vi "LIEF Example 4 - Main.vi"() -> ()   [LabVIEW 2017]
uses:
  Handler 4/Handler 4.lvclass
  C:/Program Files (x86)/National Instruments/LabVIEW 2017/vi.lib/LIEF/Image Editor Handler/Image Editor Handler.lvclass
  Cible/Cible.lvclass
  C:/Github/LIEF-Examples/LIEF Example4 - Drag&Drop/Circle/Circle.lvclass
  C:/Program Files (x86)/National Instruments/LabVIEW 2017/vi.lib/LIEF/Forms/Shape/Shape.lvclass
  <vilib>/LIEF/Image Editor Handler/Image Editor Handler.lvclass
  Circle/Circle.lvclass
  <vilib>/LIEF/Forms/Shape/Shape.lvclass
panel:
  in  "Del":bool
  in  "Boolean":bool
  out "Array":cluster{"Left":i32, "Top":i32}[](array[cluster])
  in  "Position":cluster{"Left":i32, "Top":i32}={"Left"=32, "Top"=32}
  out "Forms":picture[](array[picture])=[bytes[42], bytes[42], bytes[42], bytes[42], bytes[42], bytes[42], bytes[42], bytes[42], bytes[42], bytes[42]]
  in  "Scene":picture
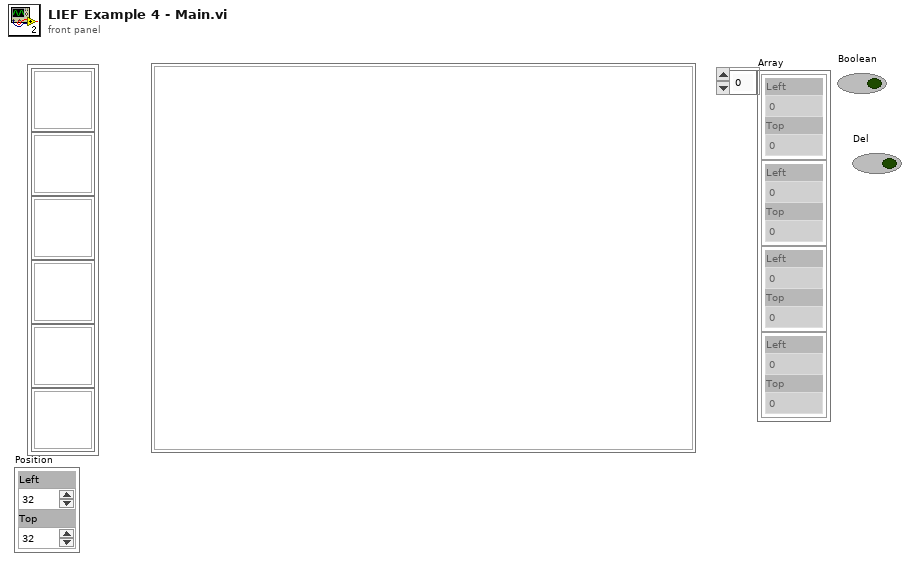
[diagram p1: front panel]
types:
  T1 = typedef "LVPoint32TypeDef.ctl" = cluster{"Horizontal":i32, "Vertical":i32}
  T2 = typedef "LVPositionTypeDef.ctl" = cluster{"Left":i32, "Top":i32}
  T3 = cluster{"data name":string, "drag data":variant}[]
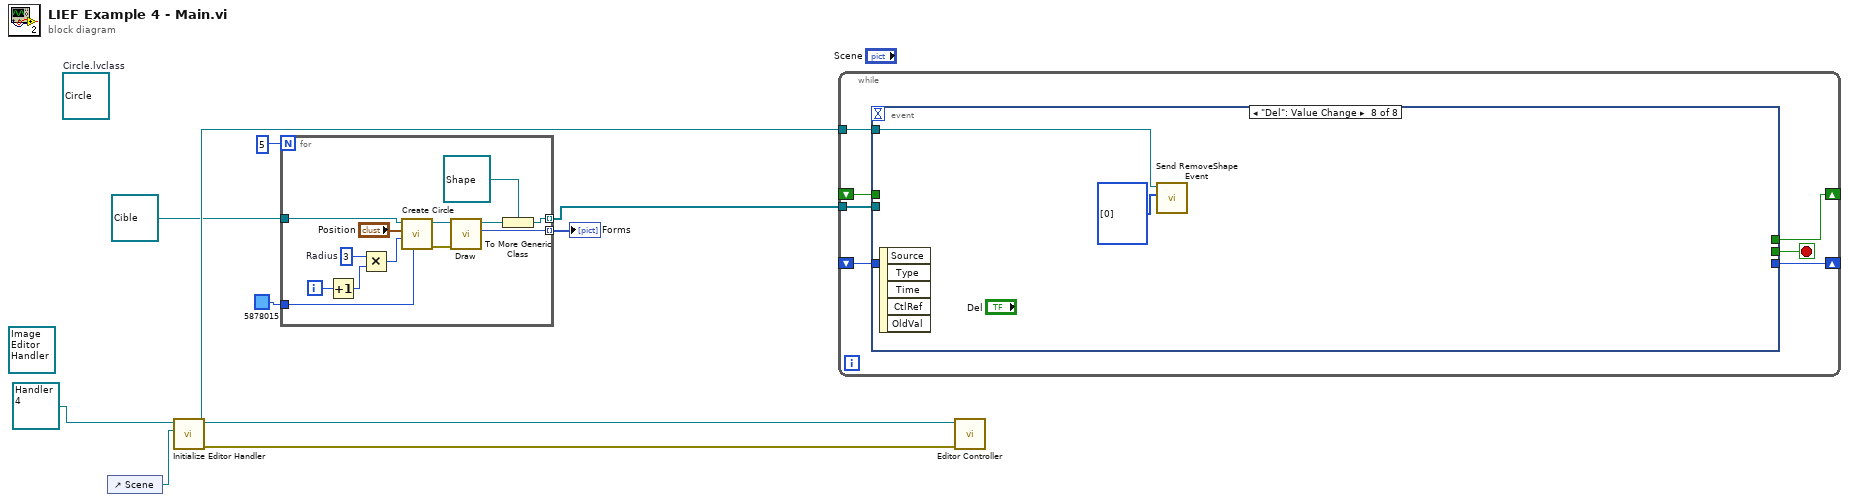
[diagram p0: block diagram]
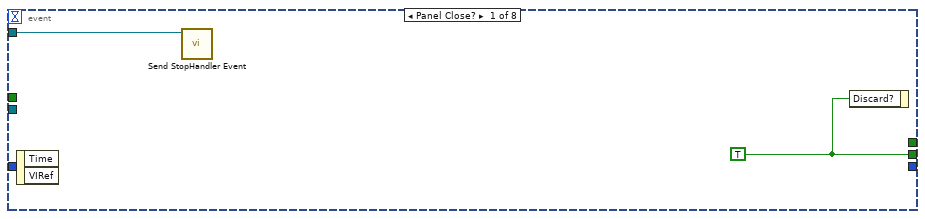
[diagram p2: hidden frame]
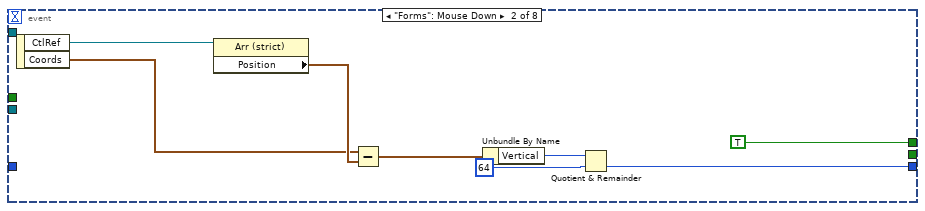
[diagram p3: hidden frame]
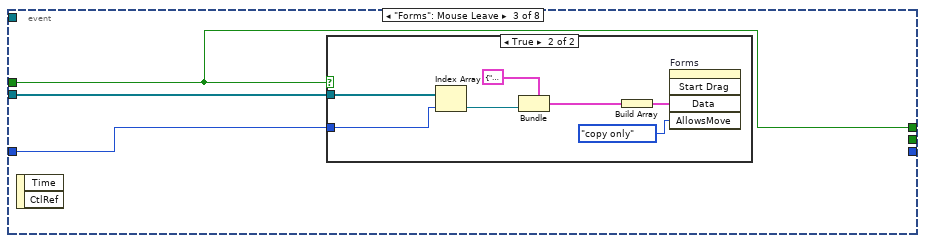
[diagram p4: hidden frame]
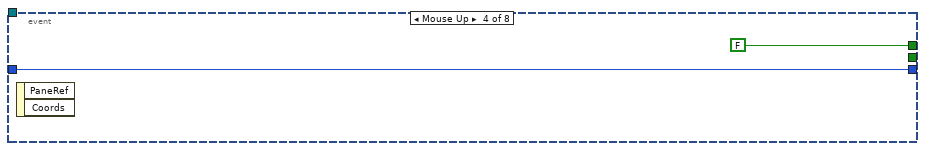
[diagram p6: hidden frame]
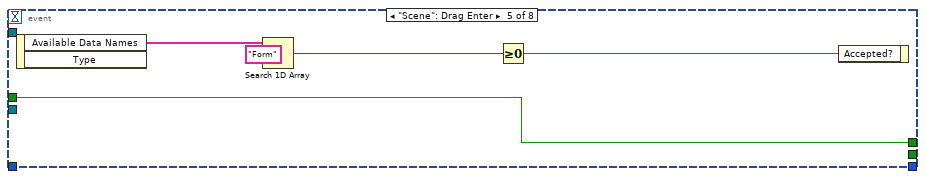
[diagram p7: hidden frame]
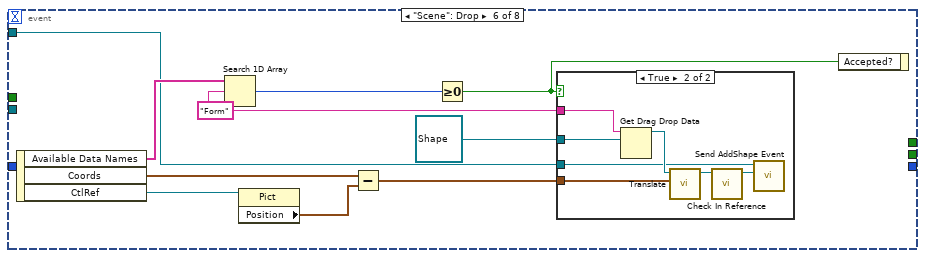
[diagram p8: hidden frame]
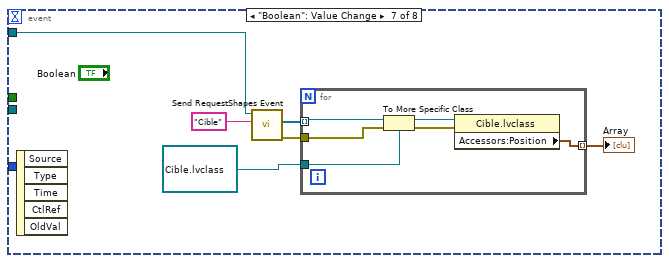
[diagram p10: hidden frame]
diagram:
  (unwired) refnum<class "Circle.lvclass"> refnum  # Circle.lvclass
  (unwired) refnum<class "Image Editor Handler.lvclass"> refnum ("Editor Handler in")
  n1 = control-ref of="Scene"() -> (w9:refnum<vi>)
  n2 = call <vilib>:"Initialize Editor Handler.vi"("PictureRef"=w9, "Editor Handler in"=refnum<class "Handler 4.lvclass"> refnum ("Handler 4.lvclass")) -> ("error out"=w7:errorcluster, "Editor Handler out"=w6:refnum<class "Handler 4.lvclass">)  [unwired: 8 in]
  n3 = for {
    N: 5 -> [_]
    tunnel: refnum<class "Cible.lvclass"> refnum ("Cible.lvclass") -> [w15]
    tunnel: u32 5878015 -> [w11]
    tunnel: [w19] -> w5 mode=indexing
    tunnel: [w20] -> w4 mode=indexing
    i -> [w22]
    w16 = 3  # Radius
    n4 = Increment(x=w22) -> (x+1=w21:i32)
    n5 = Multiply(x=w16, y=w21) -> (x*y=w12:i32)
    n6 = call "Create Circle.vi"("Color Box"=w11, "Radius"=w12, "Position"="Position", "Circle in"=w15) -> ("error out"=w10:errorcluster, "Circle out"=w14:refnum<class "Cible.lvclass">)  [unwired: 6 in]
    n7 = call-dynamic "Draw.vi"("error in (no error)"=w10, "Circle in"=w14) -> ("Picture"=w20:picture, "Circle out"=w17:refnum<class "Cible.lvclass">)  [unwired: 7 in, 1 out]
    n8 = To More Generic Class(target class=refnum<class "Shape.lvclass"> refnum ("Shape in"), reference=w17) -> (generic class reference=w19:refnum<class "Shape.lvclass">)
  }
  "Forms" <- w4
  n9 = while {
    tunnel: w6 -> [w28]
    tunnel: w5 -> [w27]
    shift-right: [w26] -> _
    shift-left: _ -> [w23]
    shift-right: [w25] -> _
    shift-left: _ -> [w24]
    stop <- w29 stop-if-true
    n10 = event shown="[7] \"Del\": Value Change" {
      selector: _ -> [_ _ _ _ _ _ _ _]
      dyn-events: _ -> [_ _ _ _ _ _ _ _]
      timeout: _ -> [_ _ _ _ _ _ _ _]
      tunnel: [w31 _ _ _ _ _ _ _] -> w29
      tunnel: w28 -> [w30 _ _ _ _ w57 w79 w86]
      tunnel: w27 -> [_ _ w42 _ _ _ _ _]
      tunnel: [_ TRUE w40 FALSE w52 _ _ _] -> w26
      tunnel: [_ w32 _ w50 _ _ _ _] -> w25
      tunnel: w24 -> [_ _ w41 w50 _ _ _ _]
      tunnel: w23 -> [_ _ w40 _ w52 _ _ _]
      event Panel Close? {
        w31 = TRUE ("Discard?")
        n11 = event-data() -> ()  [unwired: 1 in, 2 out]
        n12 = call <vilib>:"Send StopHandler Event.vi"("Editor Handler in"=w30) -> ()  [unwired: 9 in, 2 out]
        n13 = event-data("Discard?"=w31) -> ()  [unwired: 1 in, 1 out]
      }
      event "Forms": Mouse Down {
        n14 = event-data() -> ("CtlRef"=w38:refnum<vi>, "Coords"=w36:T1)  [unwired: 1 in]
        n15 = property class="Arr (strict)"(reference=w38) -> ("Position"=w37:T2)  [unwired: 1 in, 2 out]
        n16 = Subtract(x=w36, y=w37) -> (x-y=w35:T1)
        n17 = Unbundle By Name(w35) -> ("Vertical"=w34:i32)
        n18 = Quotient & Remainder(x=w34, y=64) -> (floor(x/y)=w32:i32)  [unwired: 1 out]
      }
      event "Forms": Mouse Leave {
        n19 = event-data() -> ()  [unwired: 1 in, 2 out]
        n20 = case shown="True" w40 {
          tunnel: w42 -> [_ w49]
          tunnel: w41 -> [_ w48]
          frame False {
          }
          frame True {
            n21 = Index Array(array=w49, index=w48) -> (element=w43:refnum<class "Shape.lvclass">)
            n22 = Bundle(cluster=cluster{"data name":string, "drag data":variant} {"data name"="Form", "drag data"=variant}, "drag data"=w43) -> (w45:cluster{"data name":string, "drag data":variant})  [unwired: 1 in]
            n23 = Build Array(w45) -> (w44:T3)
            n24 = invoke on="Forms" class="Arr (strict)" method="Start Drag"("Data"=w44, "AllowsMove"=enum32{"copy or move", "copy only", "move only"}."copy only" ("Drag Mode")) -> ()  [unwired: 3 in, 5 out]
          }
        }
      }
      event Mouse Up {
        n25 = event-data() -> ()  [unwired: 1 in, 2 out]
      }
      event "Scene": Drag Enter {
        n26 = event-data() -> ("Available Data Names"=w56:string[])  [unwired: 1 in, 1 out]
        n27 = Search 1D Array(1D array=w56, element="Form") -> (index of element=w54:i32)  [unwired: 1 in]
        n28 = Greater Or Equal To 0?(x=w54) -> (x >= 0?=w53:bool)
        n29 = event-data("Accepted?"=w53) -> ()  [unwired: 1 in, 1 out]
      }
      event "Scene": Drop {
        w63 = "Form" ("element")
        n30 = event-data() -> ("Available Data Names"=w66:string[], "Coords"=w60:T1, "CtlRef"=w61:refnum<vi>)  [unwired: 1 in]
        n31 = Search 1D Array(1D array=w66, element=w63) -> (index of element=w65:i32)  [unwired: 1 in]
        n32 = property class="Pict"(reference=w61) -> ("Position"=w59:T2)  [unwired: 1 in, 2 out]
        n33 = Subtract(x=w60, y=w59) -> (x-y=w58:T1)
        n34 = Greater Or Equal To 0?(x=w65) -> (x >= 0?=w64:bool)
        n35 = case shown="True" w64 {
          tunnel: w63 -> [_ w73]
          tunnel: refnum<class "Shape.lvclass"> refnum ("Shape in") -> [_ w72]
          tunnel: w58 -> [_ w70]
          tunnel: w57 -> [_ w69]
          frame False {
          }
          frame True {
            n36 = Get Drag Drop Data(8:w72, 9:w73) -> (3:w71:refnum<class "Shape.lvclass">)  [unwired: 1 in, 1 out]
            n37 = call <vilib>:"Translate.vi"("Translation"=w70, "Shape in"=w71) -> ("Shape out"=w68:refnum<class "Shape.lvclass">)  [unwired: 8 in, 1 out]
            n38 = call <vilib>:"Check In Reference.vi"("Shape in"=w68) -> ("Shape Reference"=w67:refnum<data-value>)  [unwired: 9 in, 1 out]
            n39 = call <vilib>:"Send AddShape Event.vi"("New Shape Reference"=w67, "Editor Handler in"=w69) -> ()  [unwired: 8 in, 2 out]
          }
        }
        n40 = event-data("Accepted?"=w64) -> ()  [unwired: 1 in, 1 out]
      }
      event "Boolean": Value Change {
        n41 = event-data() -> ()  [unwired: 1 in, 5 out]
        n42 = call <vilib>:"Send RequestShapes Event.vi"("Shape Class Filter"="Cible", "Editor Handler in"=w79) -> ("error out"=w77:errorcluster, "Shapes"=w76:refnum<data-value>[])  [unwired: 7 in, 1 out]
        n43 = for {
          tunnel: w77 -> [w84]
          tunnel: w76 -> [w82] mode=indexing
          tunnel: [w83] -> w75 mode=indexing
          tunnel: refnum<data-value> refnum ("Shape Reference") -> [w81]
          n44 = To More Specific Class(target class=w81, reference=w82) -> (specific class reference=w80:refnum<data-value>)  [unwired: 1 in, 1 out]
          n45 = property class="Cible.lvclass"(reference=w80, error in=w84) -> ("Accessors:Position"=w83:cluster{"Left":i32, "Top":i32})  [unwired: 2 out]
        }
        "Array" <- w75
      }
      event "Del": Value Change {
        n46 = event-data() -> ()  [unwired: 1 in, 5 out]
        n47 = call <vilib>:"Send RemoveShape Event.vi"("Indexes"=i32[] [0], "Editor Handler in"=w86) -> ()  [unwired: 8 in, 2 out]
      }
    }
  }
  n48 = call <vilib>:"Editor Controller.vi"("error in (no error)"=w7, "Editor Handler in"=w6) -> ()  [unwired: 8 in, 2 out]
